vi "Auto Elevator Set.vi"(4 "Raw Height Set":dbl, 6 "Manual Eject Piston":bool, 7 "Hold Low":bool, 8 "Force?":sgl, 9 "Command":i32, 10 "Set Idle State":i32, 11 "Mode":i32) -> ()   [LabVIEW 2014]
uses:
  Common Code/Elevator Mode.ctl
  Elevator/Elevator Command.ctl
  Common Code/Elevator Idle Mode.ctl
  Robot Global Data.vi
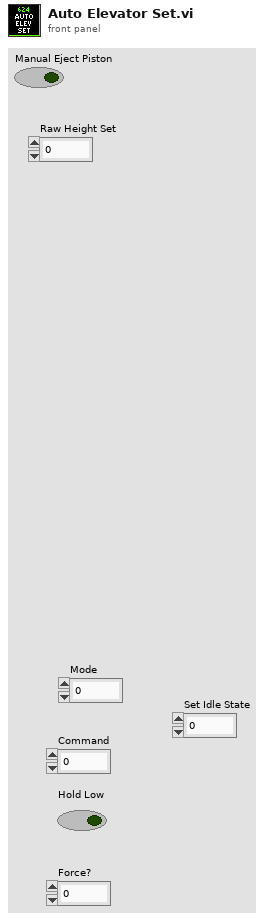
[diagram p1: front panel]
types:
  T1 = typedef "Elevator Command.ctl" = enum16{"Idle", "Load 1", "Load 2", "Load 3", "Drop Stack", "Eject Stack", "Untip Trashcan", "Load Trashcan", "HP Load", "HP Score"}
  T2 = typedef "Elevator Idle Mode.ctl" = enum16{"Load 1", "Load 2", "Load 3", "Load Can", "Untip Can", "Step Load", "Drop Stack", "Raw Height"}
  T3 = typedef "Elevator Mode.ctl" = enum16{"Manual", "Safe", "Auto"}
  T4 = typedef "Elevator Control Command.ctl" = cluster{"Command":T1, "Manual Motor Out":dbl, "Manual Eject Piston":bool, "Mode":T3, "Override Limits":bool, "Manual Stabilizer":bool, "Manual Finger":bool, "Store Trashcan?":bool, "Hold Low?":bool, "Idle Mode":T2, "HP Load":bool, "Unstick":bool, "Raw Height Set":dbl}
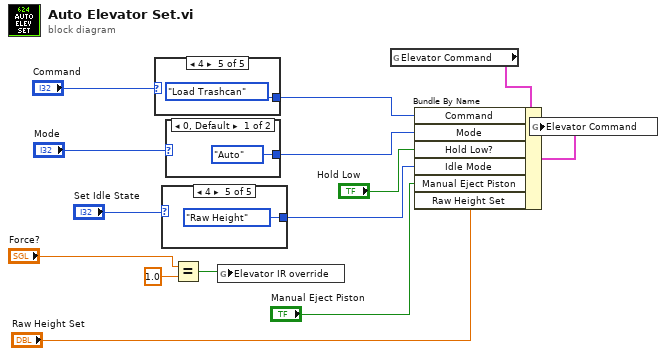
[diagram p0: block diagram]
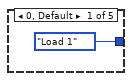
[diagram p2: hidden frame]
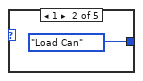
[diagram p3: hidden frame]
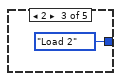
[diagram p4: hidden frame]
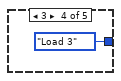
[diagram p5: hidden frame]
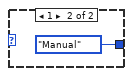
[diagram p6: hidden frame]
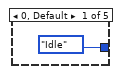
[diagram p7: hidden frame]
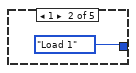
[diagram p8: hidden frame]
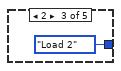
[diagram p9: hidden frame]
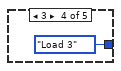
[diagram p10: hidden frame]
diagram:
  n1 = case shown="4" "Command" {
    tunnel: [Elevator_Command."Idle" ("Command") Elevator_Command."Load 1" ("Command") Elevator_Command."Load 2" ("Command") Elevator_Command."Load 3" ("Command") Elevator_Command."Load Trashcan" ("Command")] -> w13
    frame 0, Default {
    }
    frame 1 {
    }
    frame 2 {
    }
    frame 3 {
    }
    frame 4 {
    }
  }
  n2 = case shown="4" "Set Idle State" {
    tunnel: [Elevator_Idle_Mode."Load 1" ("Idle Mode") Elevator_Idle_Mode."Load Can" ("Idle Mode") Elevator_Idle_Mode."Load 2" ("Idle Mode") Elevator_Idle_Mode."Load 3" ("Idle Mode") Elevator_Idle_Mode."Raw Height" ("Idle Mode")] -> w3
    frame 0, Default {
    }
    frame 1 {
    }
    frame 2 {
    }
    frame 3 {
    }
    frame 4 {
    }
  }
  n3 = case shown="0, Default" "Mode" {
    tunnel: [Elevator_Mode."Auto" ("Mode") Elevator_Mode."Manual" ("Mode")] -> w12
    frame 0, Default {
    }
    frame 1 {
    }
  }
  n4 = Equal?(x="Force?", y=1.0) -> (x = y?=w5:bool)
  n5 = global write "Robot Global Data.vi" "Elevator IR override"(w5) -> ()
  n6 = global read "Robot Global Data.vi" "Elevator Command"() -> (w9:T4)
  n7 = Bundle By Name(cluster=w9, "Command"=w13, "Mode"=w12, "Hold Low?"="Hold Low", "Idle Mode"=w3, "Manual Eject Piston"="Manual Eject Piston", "Raw Height Set"="Raw Height Set") -> (w14:T4)
  n8 = global write "Robot Global Data.vi" "Elevator Command"(w14) -> ()
